vi "Module Main.vi"(8 "error in (no error)":errorcluster) -> (0 "error out":errorcluster)   [LabVIEW 2026, in "Error.lvlib"]
doc: "Module Main\nFor named purposes"
uses:
  Error.lvlib
  Private Control/Queue FGV Action.ctl
  Control/Control.lvlib
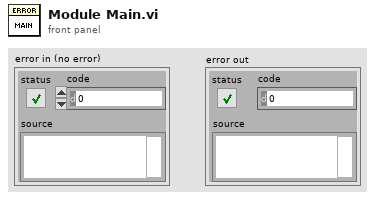
[diagram p1: front panel]
types:
  T1 = typedef "Error.lvlib/Queue FGV Action.ctl" = enum16{"Create", "Get", "Release"}
  T2 = typedef "Error.lvlib/Queue Element.ctl" = cluster{"Module Action":T3, "Data":variant}
  T3 = typedef "Error.lvlib/Module Action.ctl" = enum16{"Init", "Error Handle ", "Console Error", "Sensor IO Error", "Process Step Error", "Error Log", "Error", "Exit"}
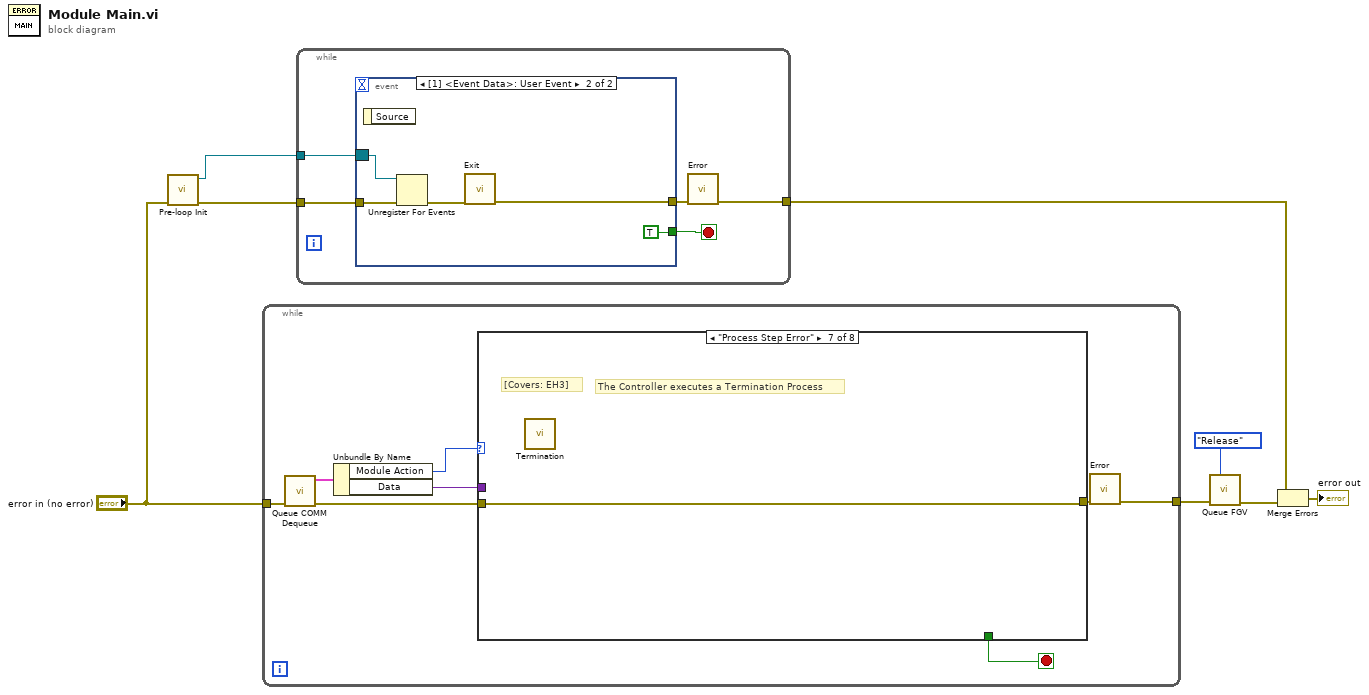
[diagram p0: block diagram]
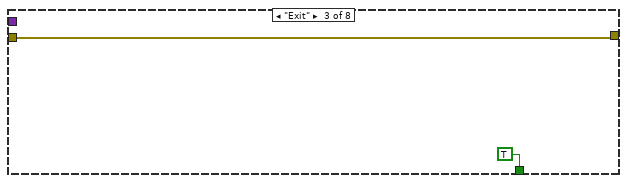
[diagram p4: hidden frame]
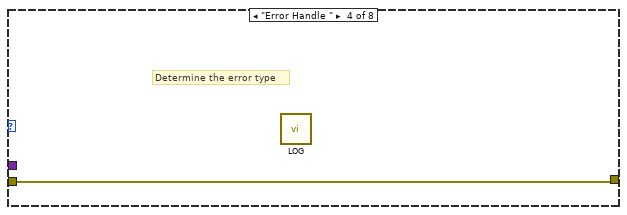
[diagram p5: hidden frame]
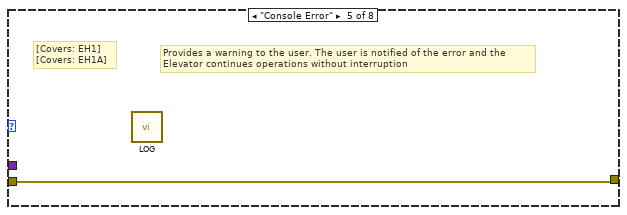
[diagram p6: hidden frame]
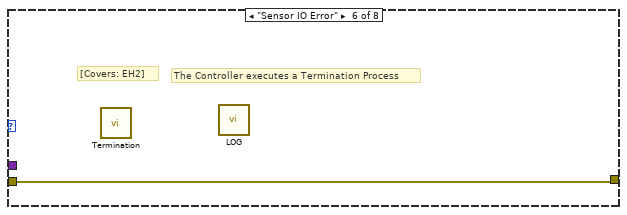
[diagram p7: hidden frame]
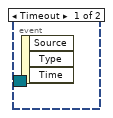
[diagram p9: hidden frame]
diagram:
  n1 = call "Pre-loop Init.vi"("error in (no error)"="error in (no error)") -> ("error out"=w7:errorcluster, "Event Registration Refnum"=w8:refnum<event-registration>)  [unwired: 9 in]
  n2 = while {
    tunnel: "error in (no error)" -> [w16]
    tunnel: [w10] -> w3
    stop <- w9 stop-if-true
    n3 = call "Queue COMM Dequeue.vi"("error in (no error)"=w16) -> ("error out"=w14:errorcluster, "element"=w15:T2)  [unwired: 9 in]
    n4 = Unbundle By Name(w15) -> ("Module Action"=w13:T3, "Data"=w12:variant)
    n5 = case shown="\"Process Step Error\"" w13 {
      tunnel: w14 -> [w17 w18 w20 w21 w22 w23 w24 w25]
      tunnel: w12 -> [_ _ _ _ _ _ _ _]
      tunnel: [w17 w18 w20 w21 w22 w23 w24 w25] -> w11
      tunnel: [_ _ TRUE _ _ _ _ _] -> w9
      frame "Init", Default {
      }
      frame "Error" {
      }
      frame "Exit" {
      }
      frame "Error Handle " {
        # "Determine the error type"
        n6 = call "LOG.vi"() -> ()  [unwired: 11 in, 1 out]
      }
      frame "Console Error" {
        # "Provides a warning to the user. The user is notified of the error and the\nElevator continues operations without interruption"
        # "[Covers: EH1] \n[Covers: EH1A]"
        n7 = call "LOG.vi"() -> ()  [unwired: 11 in, 1 out]
      }
      frame "Sensor IO Error" {
        # "The Controller executes a Termination Process"
        # "[Covers: EH2]"
        n8 = call "Termination.vi"() -> ()  [unwired: 11 in, 1 out]
        n9 = call "LOG.vi"() -> ()  [unwired: 11 in, 1 out]
      }
      frame "Process Step Error" {
        # "The Controller executes a Termination Process"
        # "[Covers: EH3]"
        n10 = call "Termination.vi"() -> ()  [unwired: 11 in, 1 out]
      }
      frame "Error Log" {
        # "[Covers: EH4]"
        # "The error handling system maintains a log file. All errors are logged with\nthe following data.\n• The error log includes a description of each error that occurs.\n• The error log includes the level of the error.\n• The error log includes the time and date at which the error occurred"
      }
    }
    n11 = call "Error.vi"("error in (no error)"=w11) -> ("error out"=w10:errorcluster)  [unwired: 10 in]
  }
  n12 = while {
    tunnel: w8 -> [w30]
    tunnel: w7 -> [w29]
    tunnel: [w27] -> w5
    stop <- w26 stop-if-true
    n13 = event shown="[1] <Event Data>: User Event" {
      selector: w30 -> [_ w34]
      dyn-events: _ -> [_ _]
      timeout: _ -> [_ _]
      tunnel: w29 -> [_ w35]
      tunnel: [_ w32] -> w28
      tunnel: [_ TRUE] -> w26
      event Timeout {
        n14 = event-data() -> ()  [unwired: 1 in, 3 out]
      }
      event User Event {
        n15 = event-data() -> ()  [unwired: 1 in, 1 out]
        n16 = Unregister For Events(event registration refnum=w34, error in=w35) -> (error out=w33:errorcluster)
        n17 = call "Exit.vi"("error in (no error)"=w33) -> ("error out"=w32:errorcluster)  [unwired: 10 in]
      }
    }
    n18 = call "Error.vi"("error in (no error)"=w28) -> ("error out"=w27:errorcluster)  [unwired: 10 in]
  }
  n19 = call "Queue FGV.vi"("error in (no error)"=w3, "Queue FGV  Action"=Queue_FGV_Action."Release") -> ("error out"=w2:errorcluster)  [unwired: 8 in, 1 out]
  n20 = Merge Errors(w5, w2) -> (→"error out":errorcluster)
